vi "Init.vi"(8 "error in (no error)":errorcluster, 11 "Data in":refnum<class "Omni_Bus.lvclass">) -> (0 "error out":errorcluster, 3 "Data out":refnum<class "Omni_Bus.lvclass">)   [LabVIEW 2021, in "Omni_Bus.lvclass"]
uses:
  Omni_Bus.lvclass
  <vilib>/TSA/Abstract Data Classes/Abs_Types/Type/Abs_Type.lvclass
  Omni_Bus.lvclass/Omni_Bus.ctl
  Bus Access/Bus_Access.lvclass/Bus_Access.ctl
  <vilib>/TSA/Abstract Data Classes/Abs_Types/Type/Abs_Type.lvclass/Abs_Type.ctl
  <vilib>/Utility/error.llb/DialogType.ctl
  Bus Access/Properties/Read Values.vi
  Bus Access/Properties/Read Tags.vi
  Properties/Read Bus Access.vi
  Properties/Write Bus Access.vi
  Properties/Write Var Map.vi
  Bus Access/Bus_Access.lvclass
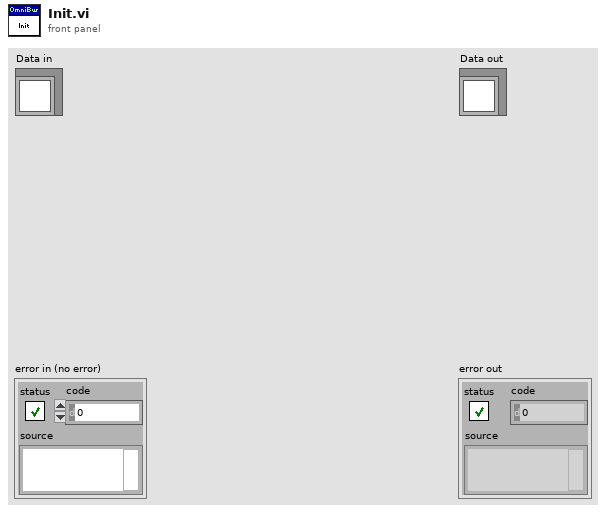
[diagram p1: front panel]
types:
  T1 = typedef "DialogType.ctl" = u16
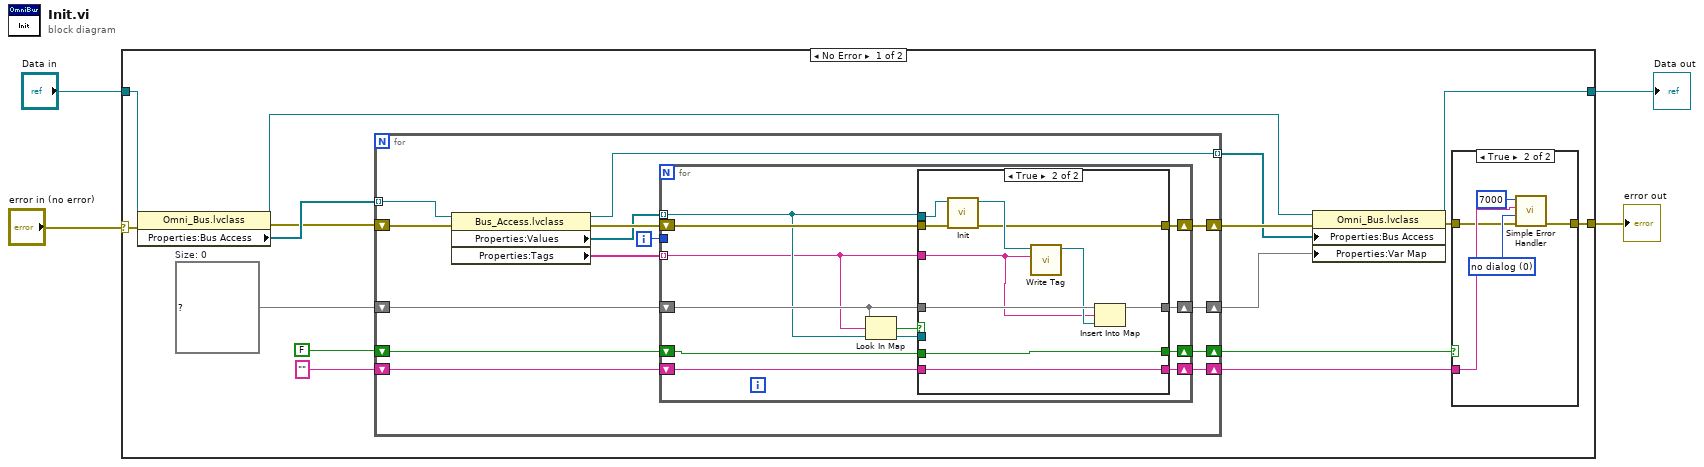
[diagram p0: block diagram]
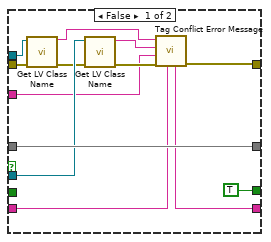
[diagram p3: hidden frame]
diagram:
  n1 = case shown="No Error" "error in (no error)" {
    selector: "error in (no error)" -> [w20 w76]
    tunnel: "Data in" -> [w19 w77]
    tunnel: [w6 w76] -> w2
    tunnel: [w13 w77] -> w1
    frame No Error {
      w12 = map{string, refnum<class "Abs_Type.lvclass">} {}  # Size: 0
      n2 = property class="Omni_Bus.lvclass"(reference=w19, error in=w20) -> (reference out=w14:refnum<class "Omni_Bus.lvclass">, error out=w17:errorcluster, "Properties:Bus Access"=w18:refnum<class "Bus_Access.lvclass">[])
      n3 = for {
        tunnel: w18 -> [w39] mode=indexing
        shift-right: [w32] -> w16
        shift-left: w17 -> [w40]
        tunnel: [w38] -> w15 mode=indexing
        shift-right: [w36] -> w11
        shift-left: w12 -> [w35]
        shift-right: [w31] -> w5
        shift-left: "" -> [w30]
        shift-right: [w29] -> w8
        shift-left: FALSE -> [w28]
        i -> [w33]
        n4 = property class="Bus_Access.lvclass"(reference=w39, error in=w40) -> (reference out=w38:refnum<class "Bus_Access.lvclass">, error out=w34:errorcluster, "Properties:Values"=w27:refnum<class "Abs_Type.lvclass">[], "Properties:Tags"=w37:string[])
        n5 = for {
          tunnel: w37 -> [w41] mode=indexing
          shift-right: [w52] -> w36
          shift-left: w35 -> [w50]
          tunnel: w33 -> [_]
          shift-right: [w48] -> w32
          shift-left: w34 -> [w51]
          shift-right: [w45] -> w31
          shift-left: w30 -> [w44]
          shift-right: [w43] -> w29
          shift-left: w28 -> [w42]
          tunnel: w27 -> [w49] mode=indexing
          n6 = Look In Map(map=w50, key=w41, default value=w49) -> (key not found?=w47:bool, value=w46:refnum<class "Abs_Type.lvclass">)
          n7 = case shown="True" w47 {
            tunnel: [w65 w75] -> w52
            tunnel: w51 -> [w63 w74]
            tunnel: w50 -> [w65 w73]
            tunnel: w41 -> [w56 w67]
            tunnel: w49 -> [w62 w72]
            tunnel: [w59 w66] -> w48
            tunnel: w46 -> [w64 _]
            tunnel: [w55 w71] -> w45
            tunnel: w44 -> [w54 w71]
            tunnel: [TRUE w70] -> w43
            tunnel: w42 -> [_ w70]
            frame False {
              n8 = call <vilib>:"Get LV Class Name.vi"("error in (no error)"=w63, "object"=w62) -> ("error out"=w61:errorcluster, "class name"=w58:string)  [unwired: 8 in]
              n9 = call <vilib>:"Get LV Class Name.vi"("error in (no error)"=w61, "object"=w64) -> ("error out"=w60:errorcluster, "class name"=w57:string)  [unwired: 8 in]
              n10 = call "Tag Conflict Error Message.vi"("Previous Error Message"=w54, "error in (no error)"=w60, "Tag Name"=w56, "Conflict Class"=w57, "Original Class"=w58) -> ("error out"=w59:errorcluster, "Error Message"=w55:string)  [unwired: 5 in]
            }
            frame True {
              n11 = call-dynamic "Init.vi"("error in (no error)"=w74, "Data in"=w72) -> ("error out"=w66:errorcluster, "Data out"=w69:refnum<class "Abs_Type.lvclass">)  [unwired: 8 in]
              n12 = call <vilib>:"Write Tag.vi"("Tag"=w67, "Abs_Type in"=w69) -> ("Abs_Type out"=w68:refnum<class "Abs_Type.lvclass">)  [unwired: 9 in]
              n13 = Insert Into Map(map in=w73, key=w67, value=w68) -> (map out=w75:map{string, refnum<class "Abs_Type.lvclass">})  [unwired: 2 out]
            }
          }
        }
      }
      n14 = property class="Omni_Bus.lvclass"(reference=w14, error in=w16, "Properties:Bus Access"=w15, "Properties:Var Map"=w11) -> (reference out=w13:refnum<class "Omni_Bus.lvclass">, error out=w7:errorcluster)
      n15 = case shown="True" w8 {
        tunnel: w7 -> [w21 w22]
        tunnel: [w21 w26] -> w6
        tunnel: w5 -> [_ w23]
        frame False {
        }
        frame True {
          w25 = T1 0 items=["no dialog", "OK message", "continue or stop message", "OK message + warnings", "continue/stop + warnings"] ("type of dialog (OK msg:1)")
          n16 = call <vilib>:"Simple Error Handler.vi"("error code (no error:0)"=7000, "error source (\" \")"=w23, "type of dialog (OK msg:1)"=w25, "error in (no error)"=w22) -> ("error out"=w26:errorcluster)  [unwired: 1 in, 4 out]
        }
      }
    }
    frame Error {
    }
  }
  "error out" <- w2
  "Data out" <- w1
